vi "Program list Selection.vi"(8 "error in":errorcluster, 10 "Filepath":path=path "D:/My Project/2019-2020/Magnetic Mareli UM/MM_UM/Project Setup/data/program seq/Program_280A.bin", 11 "vi referenceIn":refnum<vi>) -> (0 "error out":errorcluster, 1 "Exit":bool, 2 "String":string, 3 "vi reference Out":refnum<vi>)   [LabVIEW 2015]
uses:
  Control Button/Exit.ctl
  Control Button/next.ctl
  Galobal variable_TI.vi
  <vilib>/addons/database/Connection.llb/DB Tools Open Connec (String).vi
  <vilib>/addons/database/_DB Variant To Data/Database Variant To Data.xnode
  <vilib>/addons/database/NI_Database_API.lvlib
panel:
  out "error out 3":errorcluster
  out "error out 2":errorcluster
  out "String 2":string
  in  "Next":T1
  in  "Exit":T2
  in  "Program List":string(combo)
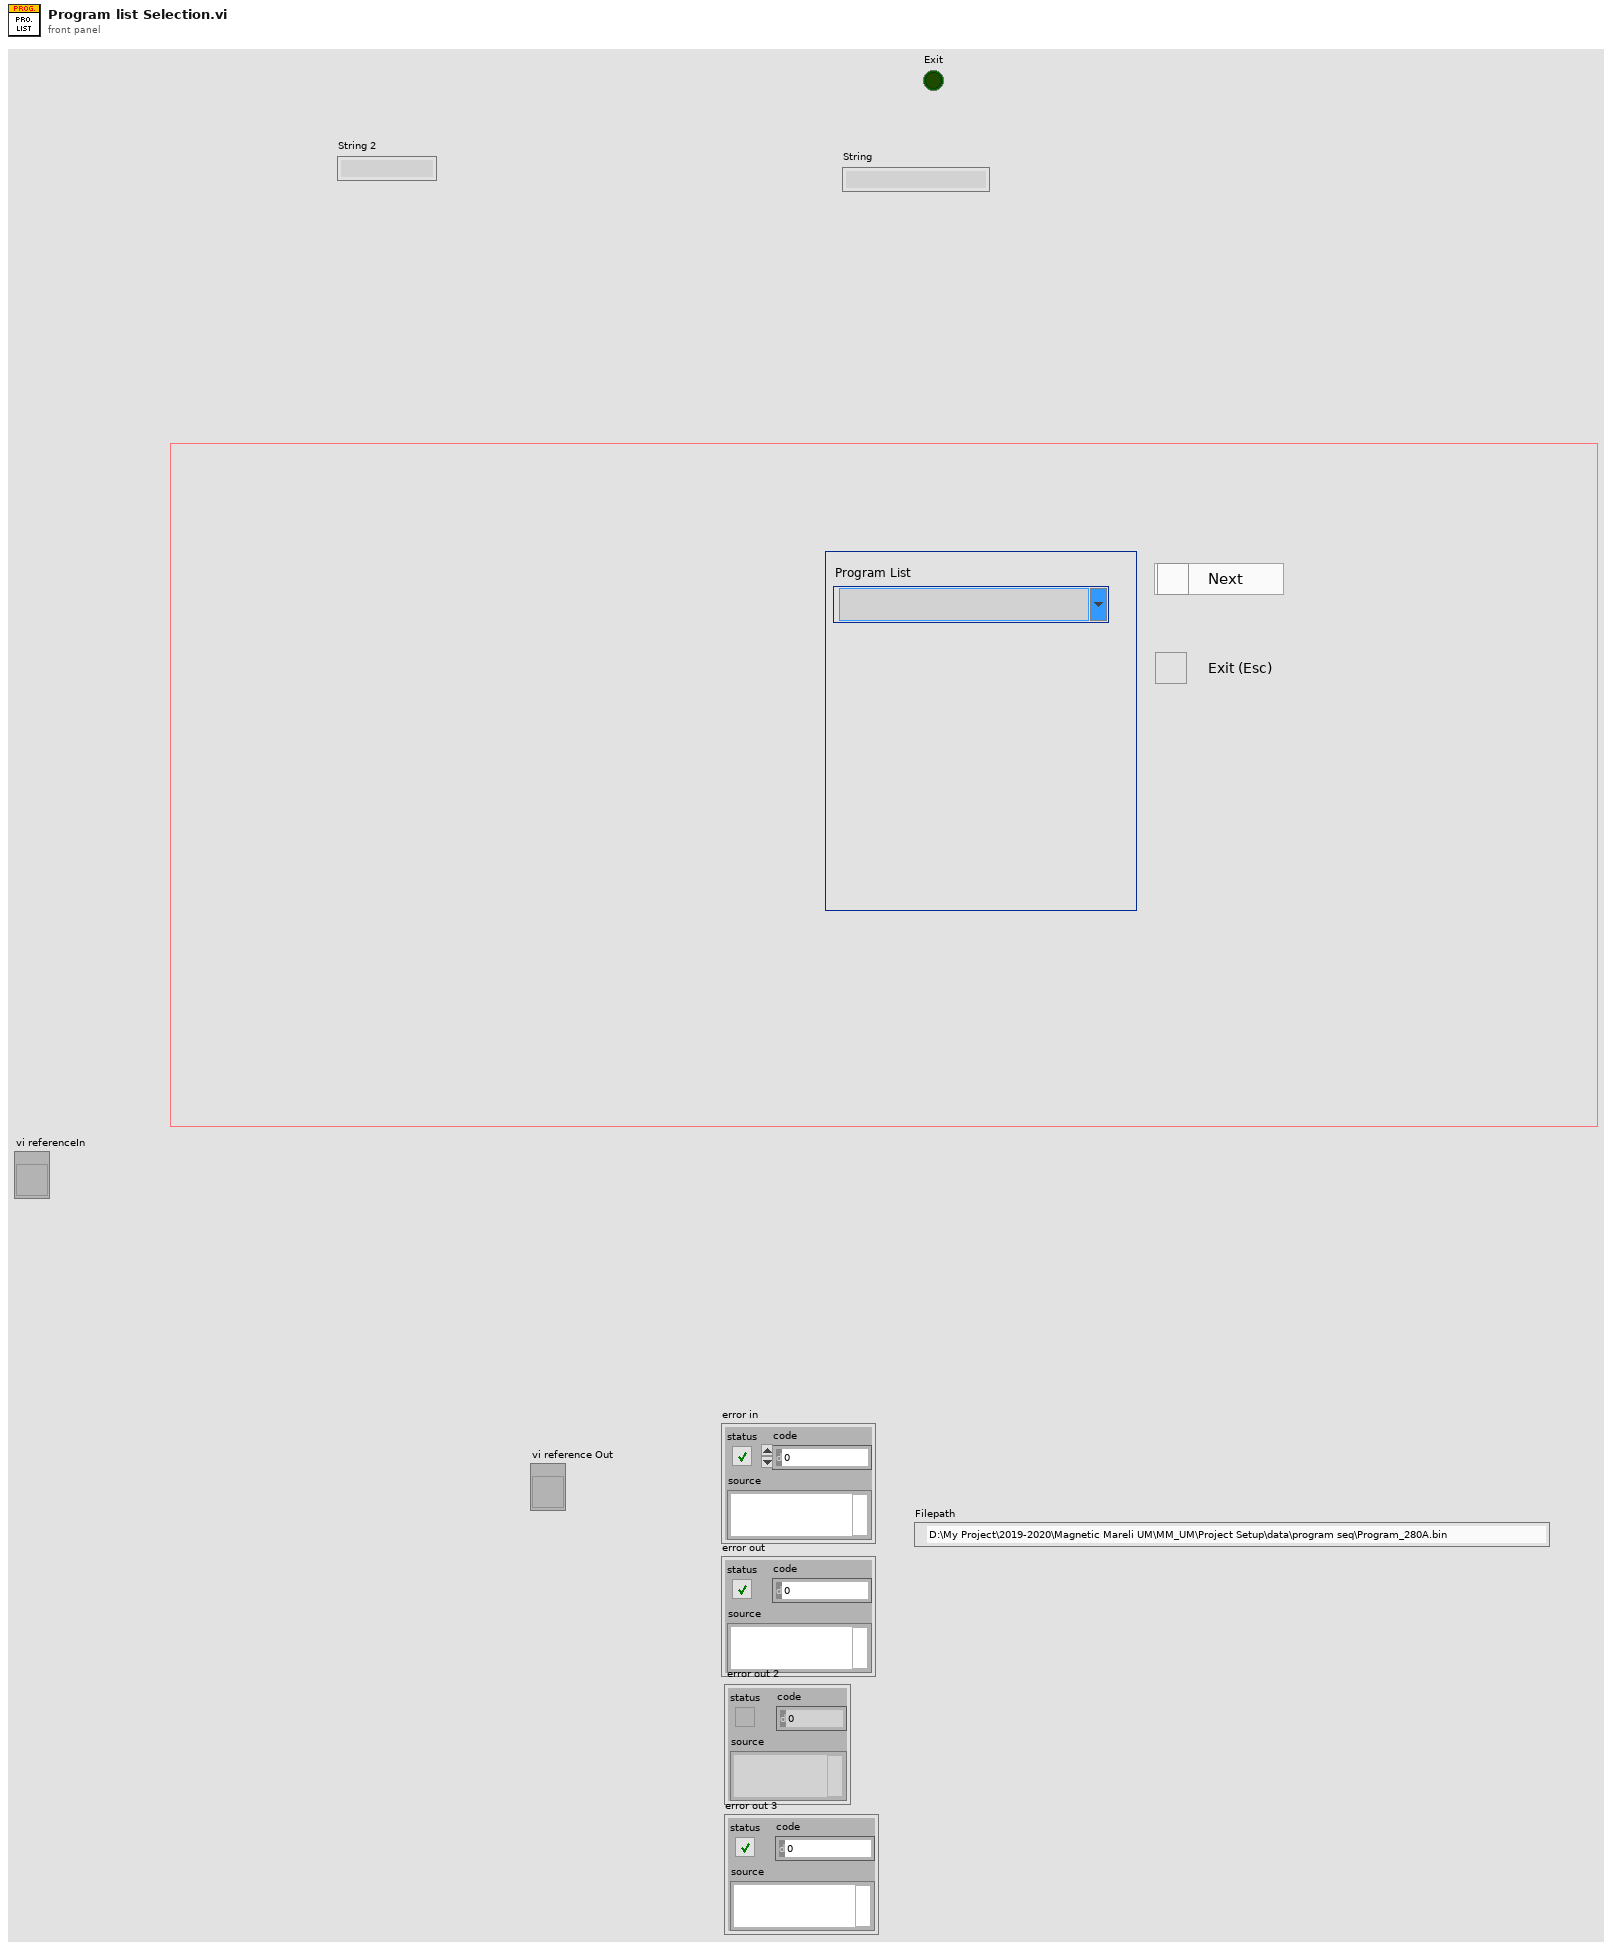
[diagram p1: front panel]
types:
  T1 = typedef "next.ctl" = bool
  T2 = typedef "Exit.ctl" = bool
  T3 = cluster{"MaxLoad(N) ":dbl, "Min Load(N)":dbl, "Load Offset":dbl, "Model":string, "MIC Code":string, "Dailcode1":string, "Dailcode2":string, "DailStrip1":string, "DailStrip2":string}
  T4 = enum32{"Invalid", "Standard", "Closed", "Hidden", "Minimized", "Maximized"}
  T5 = typedef "NI_Database_API.lvlib/Conn ObjectReference.ctl" = refnum<k1>
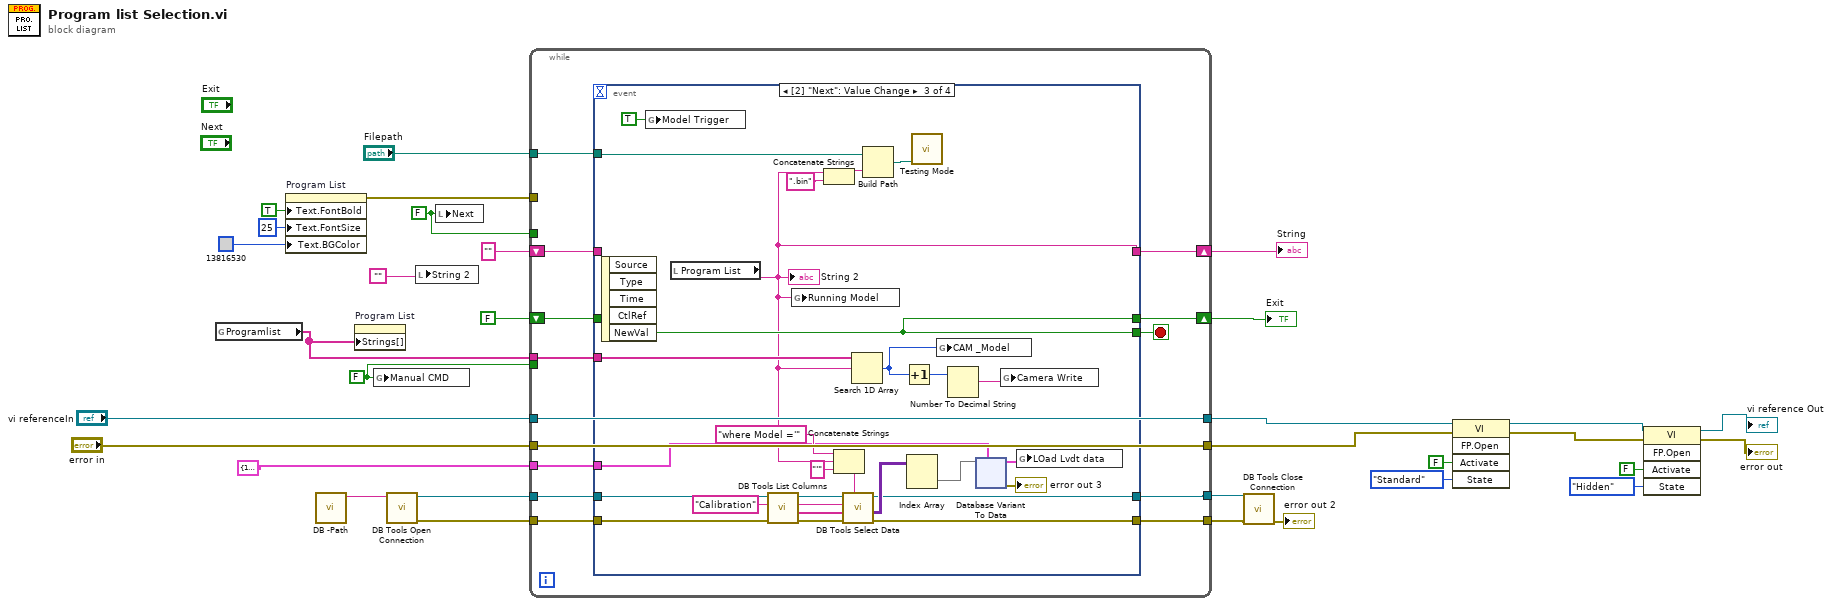
[diagram p0: block diagram]
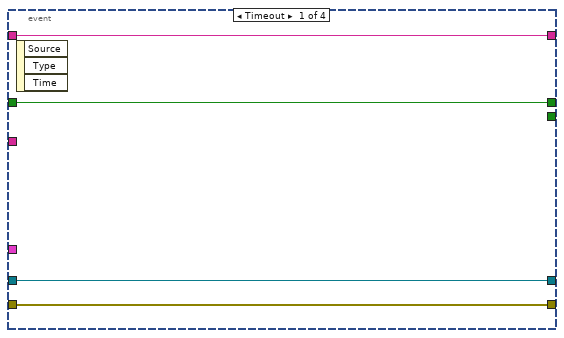
[diagram p2: hidden frame]
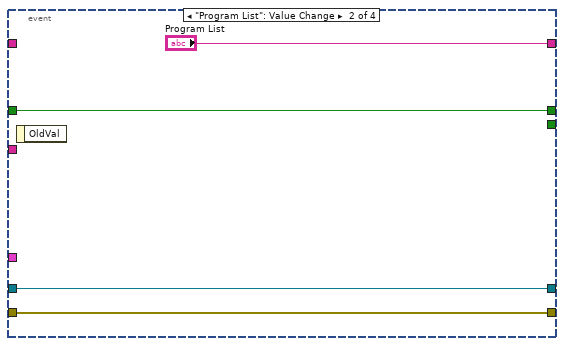
[diagram p3: hidden frame]
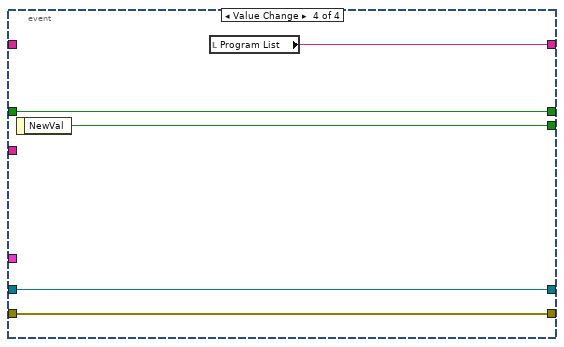
[diagram p4: hidden frame]
diagram:
  w21 = FALSE ("Manual CMD")
  w22 = FALSE ("Next")
  n1 = global read "Galobal variable_TI.vi" "Programlist"() -> (w28:string[])
  n2 = property on="Program List" class="CmbBox"("Text.FontBold"=TRUE ("Text.Font:Bold"), "Text.FontSize"=u32 25 ("Text.Font:Size"), "Text.BGColor"=u32 13816530 ("Color Box")) -> (error out=w25:errorcluster)  [unwired: 2 in, 1 out]
  n3 = call "DB -Path.vi"() -> ("String"=w19:string)  [unwired: 11 in]
  n4 = property on="Program List" class="CmbBox"("Strings[]"=w28) -> ()  [unwired: 2 in, 2 out]
  n5 = global write "Galobal variable_TI.vi" "Manual CMD"(w21) -> ()
  n6 = call-poly <vilib>:"DB Tools Open Connection.vi"("connection information"=w19) -> ("error out"=w17:errorcluster, "connection reference"=w18:T5)  [unwired: 7 in]
  n7 = local write "String 2"("") -> ()
  n8 = local write "Next"(w22) -> ()
  n9 = while {
    shift-right: [w46] -> w32
    shift-left: "" ("Combo Box") -> [w45]
    shift-right: [w43] -> w29
    shift-left: T2 FALSE ("NewVal") -> [w42]
    tunnel: w28 -> [w33]
    tunnel: w25 -> [_]
    tunnel: w22 -> [_]
    tunnel: w21 -> [_]
    tunnel: "vi referenceIn" -> [w41]
    tunnel: [w41] -> w5
    tunnel: "error in" -> [w40]
    tunnel: [w40] -> w4
    tunnel: "Filepath" -> [w39]
    tunnel: w18 -> [w38]
    tunnel: w17 -> [w37]
    tunnel: [w36] -> w16
    tunnel: [w35] -> w15
    tunnel: T3 {"MaxLoad(N) "=1.0, "Min Load(N)"=2.0, "Load Offset"=3.0, "Model"="Medium", "MIC Code"="05487", "Dailcode1"="AAEPL29", "Dailcode2"="AAEPL29A", "DailStrip1"="AAEPL29B", "DailStrip2"="AAEPL29C"} ("LOad Lvdt data") -> [w34]
    stop <- w44 stop-if-true
    n10 = event shown="[2] \"Next\": Value Change" {
      selector: _ -> [_ _ _ _]
      dyn-events: _ -> [_ _ _ _]
      timeout: _ -> [_ _ _ _]
      tunnel: [w50 "Program List" w56 w368] -> w46
      tunnel: w45 -> [w50 _ _ _]
      tunnel: [_ _ w81 w369] -> w44
      tunnel: [w49 w53 w81 w367] -> w43
      tunnel: w42 -> [w49 w53 _ w367]
      tunnel: w39 -> [_ _ w78 _]
      tunnel: w38 -> [w48 w52 w67 w366]
      tunnel: w37 -> [w47 w51 w66 w365]
      tunnel: [w48 w52 w65 w366] -> w36
      tunnel: [w47 w51 w64 w365] -> w35
      tunnel: w34 -> [_ _ w62 _]
      tunnel: w33 -> [_ _ w60 _]
      event Timeout {
        n11 = event-data() -> ()  [unwired: 1 in, 3 out]
      }
      event "Program List": Value Change {
        n12 = event-data() -> ()  [unwired: 1 in, 1 out]
      }
      event Value Change {
        w73 = "Calibration" ("table")
        n13 = event-data() -> ("NewVal"=w81:T1)  [unwired: 1 in, 4 out]
        n14 = global write "Galobal variable_TI.vi" "Model Trigger"(TRUE ("Model Trigger")) -> ()
        n15 = local read "Program List"() -> (w56:string)
        "String 2" <- w56
        n16 = call <vilib>:"DB Tools List Columns.vi"("error in (no error)"=w66, "table"=w73, "connection reference"=w67) -> ("error out"=w70:errorcluster, "columns"=w72:string[], "connection reference out"=w71:T5)  [unwired: 1 in, 1 out]
        n17 = global write "Galobal variable_TI.vi" "Running Model"(w56) -> ()
        n18 = Concatenate Strings(w56, ".bin" ("string")) -> (w79:string)
        n19 = Concatenate Strings("where Model ='" ("string"), w56, "'" ("string")) -> (w69:string)
        n20 = call <vilib>:"DB Tools Select Data.vi"("condition"=w69, "error in (no error)"=w70, "columns"=w72, "table"=w73, "connection reference"=w71) -> ("error out"=w64:errorcluster, "data"=w68:variant[][], "connection reference out"=w65:T5)  [unwired: 1 in]
        n21 = Search 1D Array(1D array=w60, element=w56) -> (index of element=w55:i32)  [unwired: 1 in]
        n22 = Build Path(base path=w78, name or relative path=w79) -> (appended path=w77:path)
        n23 = Increment(x=w55) -> (x+1=w59:i32)
        n24 = Index Array(array=w68) -> (element=w76:variant[])  [unwired: 2 in]
        n25 = call "Testing Mode.vi"("Filepath"=w77) -> ()  [unwired: 9 in, 1 out]
        n26 = global write "Galobal variable_TI.vi" "CAM _Model"(w55) -> ()
        n27 = Number To Decimal String(number=w59) -> (decimal integer string=w58:string)  [unwired: 1 in]
        n28 = xnode "Database Variant To Data"("database variant"=w76, "type"=w62) -> ("data"=w61:T3, "error out"=→"error out 3":errorcluster)  [unwired: 1 in]
        n29 = global write "Galobal variable_TI.vi" "Camera Write"(w58) -> ()
        n30 = global write "Galobal variable_TI.vi" "LOad Lvdt data"(w61) -> ()
      }
      event Value Change {
        n31 = event-data() -> ("NewVal"=w369:T2)  [unwired: 1 in]
        n32 = local read "Program List"() -> (w368:string)
      }
    }
  }
  "String" <- w32
  "Exit" <- w29
  n33 = call <vilib>:"DB Tools Close Connection.vi"("error in (no error)"=w15, "connection reference"=w16) -> ("error out"=→"error out 2":errorcluster)  [unwired: 5 in]
  n34 = invoke class="VI" method="FP.Open"(reference=w5, error in=w4, "Activate"=FALSE ("Activate?"), "State"=T4."Standard") -> (reference out=w7:refnum<vi>, error out=w6:errorcluster)  [unwired: 1 in, 3 out]
  n35 = invoke class="VI" method="FP.Open"(reference=w7, error in=w6, "Activate"=FALSE ("Activate?"), "State"=T4."Hidden") -> (reference out=→"vi reference Out":refnum<vi>, error out=→"error out":errorcluster)  [unwired: 1 in, 3 out]
